vi "BMark_Get VIs in Project.vi"(8 "error in (no error)":errorcluster, 11 "project":refnum<vi>) -> (0 "error out":errorcluster, 2 "Array of VIs":T1[](array[typedef]), 3 "project out":refnum<vi>)   [LabVIEW 2018]
uses:
  controls/BMark_VI_Identifier.ctl
  <vilib>/addons/analyzer/_analyzerctrls.llb/VIAnCtl Analysis App Info.ctl
panel:
  out "Libraries":T1[][](array[typedef])
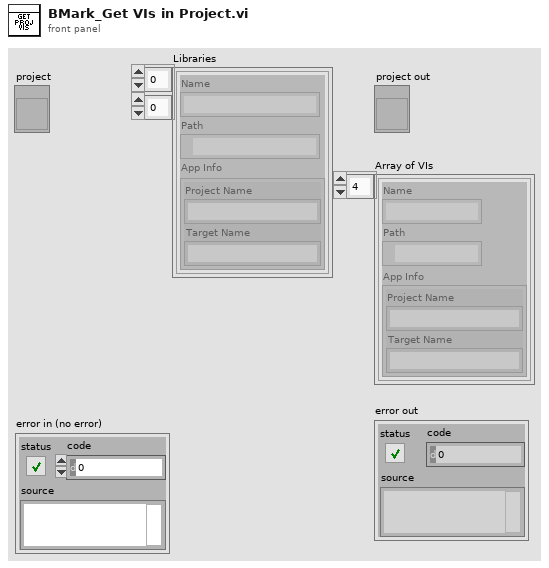
[diagram p1: front panel]
types:
  T1 = typedef "BMark_VI_Identifier.ctl" = cluster{"Name":string, "Path":path, "App Info":T2}
  T2 = typedef "VIAnCtl Analysis App Info.ctl" = cluster{"Project Name":string, "Target Name":string}
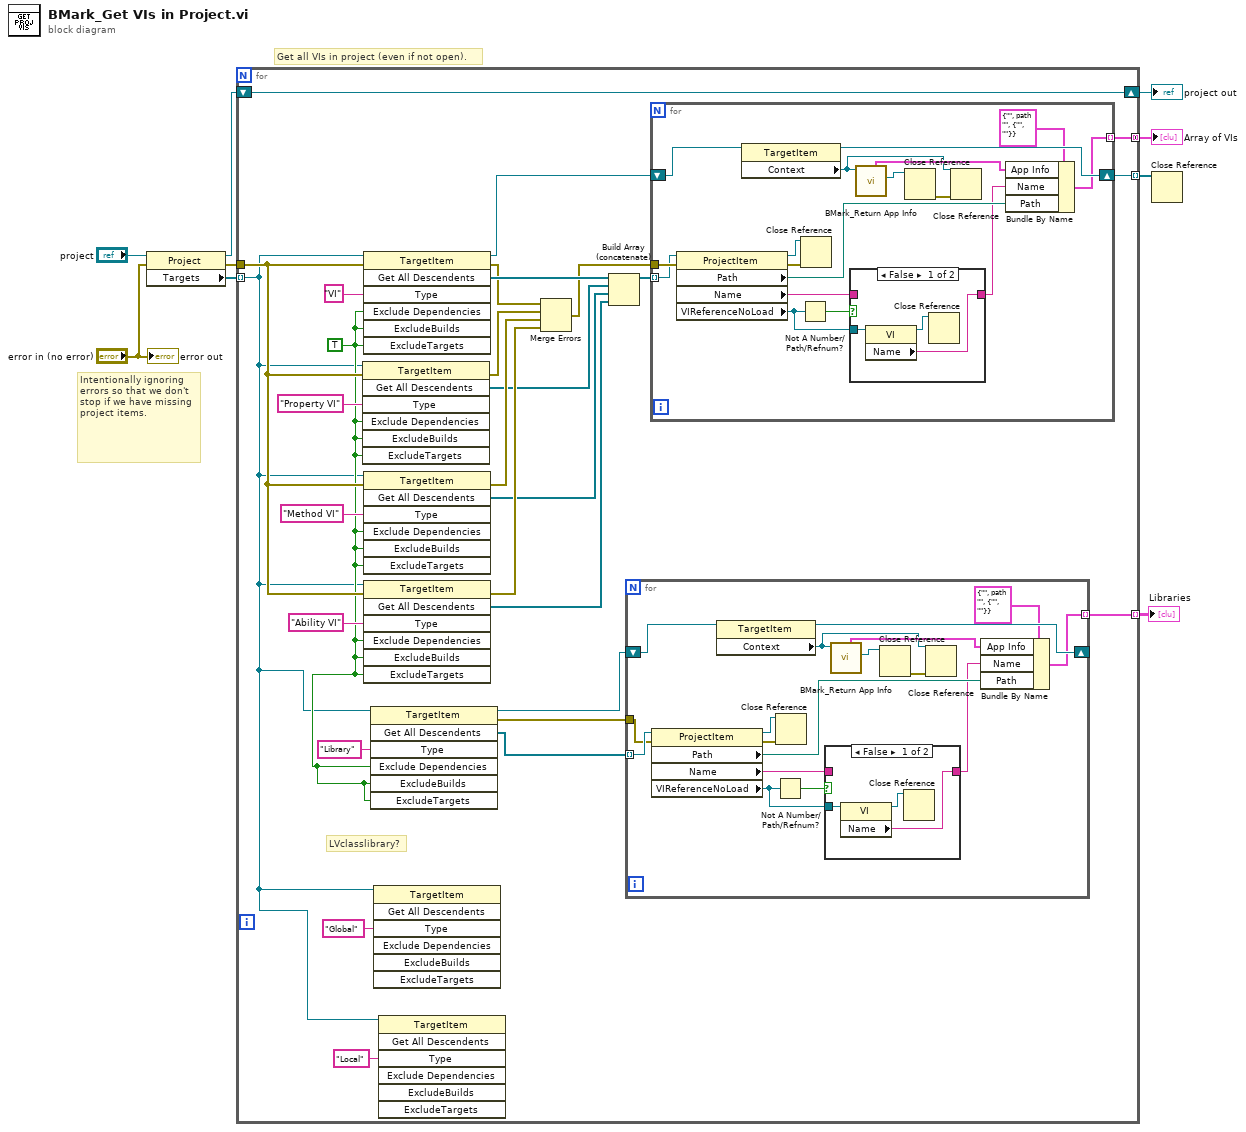
[diagram p0: block diagram]
diagram:
  # "Intentionally ignoring errors so that we don't stop if we have missing project items."
  # "Get all VIs in project (even if not open)."
  n1 = property class="Project"(reference="project", error in="error in (no error)") -> (reference out=w3:refnum<vi>, error out=w7:errorcluster, "Targets"=w9:refnum<vi>[])
  n2 = for {
    tunnel: w9 -> [w10] mode=indexing
    tunnel: [w35] -> w6 mode=indexing
    tunnel: [w34] -> w5 mode=concatenating
    tunnel: w7 -> [w26]
    shift-right: [w33] -> w2
    shift-left: w3 -> [w33]
    tunnel: [w13] -> w1 mode=indexing
    w17 = TRUE ("ExcludeDependencies")
    # "LVclasslibrary?"
    n3 = invoke class="TargetItem" method="Get All Descendents"(reference=w10, error in=w26, "Type"="Property VI", "Exclude Dependencies"=w17, "ExcludeBuilds"=w17, "ExcludeTargets"=w17) -> (error out=w25:errorcluster, "All Descendents"=w21:refnum<vi>[])  [unwired: 1 in, 5 out]
    n4 = invoke class="TargetItem" method="Get All Descendents"(reference=w10, error in=w26, "Type"="VI", "Exclude Dependencies"=w17, "ExcludeBuilds"=w17, "ExcludeTargets"=w17) -> (reference out=w36:refnum<vi>, error out=w31:errorcluster, "All Descendents"=w37:refnum<vi>[])  [unwired: 1 in, 4 out]
    n5 = invoke class="TargetItem" method="Get All Descendents"(reference=w10, error in=w26, "Type"="Method VI", "Exclude Dependencies"=w17, "ExcludeBuilds"=w17, "ExcludeTargets"=w17) -> (error out=w24:errorcluster, "All Descendents"=w20:refnum<vi>[])  [unwired: 1 in, 5 out]
    n6 = invoke class="TargetItem" method="Get All Descendents"(reference=w10, error in=w26, "Type"="Ability VI", "Exclude Dependencies"=w17, "ExcludeBuilds"=w17, "ExcludeTargets"=w17) -> (error out=w23:errorcluster, "All Descendents"=w19:refnum<vi>[])  [unwired: 1 in, 5 out]
    n7 = invoke class="TargetItem" method="Get All Descendents"(reference=w10, "Type"="Library", "Exclude Dependencies"=w17, "ExcludeBuilds"=w17, "ExcludeTargets"=w17) -> (reference out=w14:refnum<vi>, error out=w15:errorcluster, "All Descendents"=w16:refnum<vi>[])  [unwired: 2 in, 4 out]
    n8 = invoke class="TargetItem" method="Get All Descendents"(reference=w10, "Type"="Global") -> ()  [unwired: 5 in, 7 out]
    n9 = invoke class="TargetItem" method="Get All Descendents"(reference=w10, "Type"="Local") -> ()  [unwired: 5 in, 7 out]
    n10 = Merge Errors(w31, w25, w24, w23) -> (w30:errorcluster)
    n11 = Build Array (concatenate)(w37, w21, w20, w19) -> (w22:refnum<vi>[])
    n12 = for {
      tunnel: w16 -> [w41] mode=indexing
      shift-right: [w52] -> _
      shift-left: w14 -> [w39]
      tunnel: [w49] -> w13 mode=indexing
      tunnel: w15 -> [w38]
      n13 = property class="ProjectItem"(reference=w41, error in=w38) -> (reference out=w53:refnum<vi>, error out=w54:errorcluster, "Path"=w50:path, "Name"=w47:string, "VIReferenceNoLoad"=w40:refnum<vi>)
      n14 = property class="TargetItem"(reference=w39) -> (reference out=w52:refnum<vi>, "Context"=w42:refnum<vi>)  [unwired: 1 in, 1 out]
      n15 = Not A Number/Path/Refnum?(number/path/refnum=w40) -> (NaN/Path/Refnum?=w48:bool)
      n16 = Close Reference(reference=w53, error in (no error)=w54) -> ()  [unwired: 1 out]
      n17 = case shown="False" w48 {
        tunnel: w47 -> [_ w58]
        tunnel: [w56 w58] -> w46
        tunnel: w40 -> [w57 _]
        frame False {
          n18 = property class="VI"(reference=w57) -> (reference out=w55:refnum<vi>, "Name"=w56:string)  [unwired: 1 in, 1 out]
          n19 = Close Reference(reference=w55) -> ()  [unwired: 1 in, 1 out]
        }
        frame True {
        }
      }
      n20 = call "BMark_Return App Info.vi"("App Refnum in"=w42) -> ("App Refnum for Opening VI"=w44:refnum<vi>, "App Info"=w45:T2)  [unwired: 8 in, 1 out]
      n21 = Close Reference(reference=w44) -> (error out=w43:errorcluster)  [unwired: 1 in]
      n22 = Close Reference(reference=w42, error in (no error)=w43) -> ()  [unwired: 1 out]
      n23 = Bundle By Name(cluster=T1 {"Name"="", "Path"=path "", "App Info"={"Project Name"="", "Target Name"=""}}, "App Info"=w45, "Name"=w46, "Path"=w50) -> (w49:T1)
    }
    n24 = for {
      tunnel: w22 -> [w61] mode=indexing
      shift-right: [w72] -> w35
      shift-left: w36 -> [w59]
      tunnel: [w69] -> w34 mode=indexing
      tunnel: w30 -> [w75]
      n25 = property class="ProjectItem"(reference=w61, error in=w75) -> (reference out=w73:refnum<vi>, error out=w74:errorcluster, "Path"=w70:path, "Name"=w67:string, "VIReferenceNoLoad"=w60:refnum<vi>)
      n26 = property class="TargetItem"(reference=w59) -> (reference out=w72:refnum<vi>, "Context"=w62:refnum<vi>)  [unwired: 1 in, 1 out]
      n27 = Not A Number/Path/Refnum?(number/path/refnum=w60) -> (NaN/Path/Refnum?=w68:bool)
      n28 = Close Reference(reference=w73, error in (no error)=w74) -> ()  [unwired: 1 out]
      n29 = case shown="False" w68 {
        tunnel: w67 -> [_ w79]
        tunnel: [w77 w79] -> w66
        tunnel: w60 -> [w78 _]
        frame False {
          n30 = property class="VI"(reference=w78) -> (reference out=w76:refnum<vi>, "Name"=w77:string)  [unwired: 1 in, 1 out]
          n31 = Close Reference(reference=w76) -> ()  [unwired: 1 in, 1 out]
        }
        frame True {
        }
      }
      n32 = call "BMark_Return App Info.vi"("App Refnum in"=w62) -> ("App Refnum for Opening VI"=w64:refnum<vi>, "App Info"=w65:T2)  [unwired: 8 in, 1 out]
      n33 = Close Reference(reference=w64) -> (error out=w63:errorcluster)  [unwired: 1 in]
      n34 = Close Reference(reference=w62, error in (no error)=w63) -> ()  [unwired: 1 out]
      n35 = Bundle By Name(cluster=T1 {"Name"="", "Path"=path "", "App Info"={"Project Name"="", "Target Name"=""}}, "App Info"=w65, "Name"=w66, "Path"=w70) -> (w69:T1)
    }
  }
  "Array of VIs" <- w5
  "project out" <- w2
  "Libraries" <- w1
  n36 = Close Reference(reference=w6) -> ()  [unwired: 1 in, 1 out]
  "error out" <- "error in (no error)"
